vi "EZ Resistance.vi"(6 "2w/4w (F:2w)":bool, 7 "Scan List (empty)":string, 8 "error in (no error)":errorcluster, 9 "Range (7:Auto)":T2(ring)=enum."Auto", 10 "Resolution (5:Default)":T1(ring)=enum."Default", 11 "VISA Resource Name":refnum<visa-resource-name>) -> (0 "error out":errorcluster, 2 "Output Array":dbl[](array[numeric]) format="%.2f", 3 "VISA Resource Name Out":refnum<visa-resource-name>)   [LabVIEW 2017, in "Agilent 34970.lvlib"]
doc: "This VI allows you to take simple resistance measurements (either 2-wire or 4-wire)."
uses:
  <instrlib>/Agilent 34970/Agilent 34970.lvlib
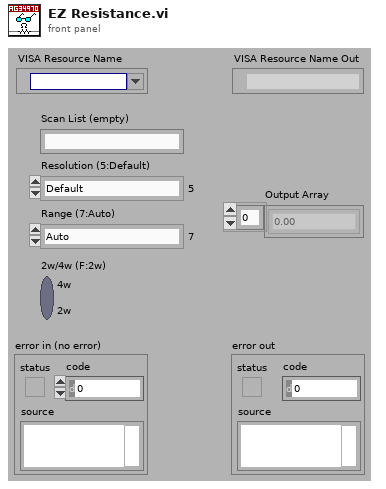
[diagram p1: front panel]
types:
  T1 = enum16{"4 1/2", "5 1/2", "6 1/2", "Least", "Highest", "Default"}
  T2 = enum16{"100 Ohm", "1 kOhm", "10 kOhm", "100 kOhm", "1 MOhm", "10 MOhm", "100 MOhm", "Auto", "Minimum", "Maximum"}
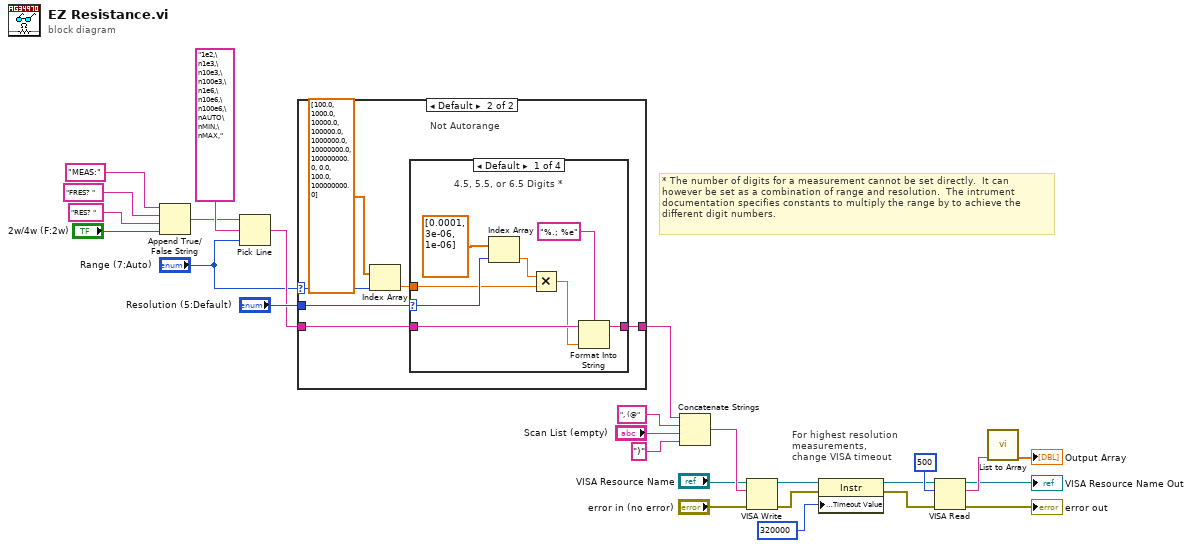
[diagram p0: block diagram]
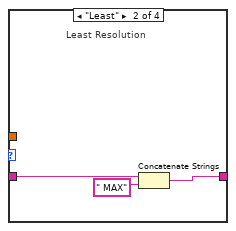
[diagram p3: hidden frame]
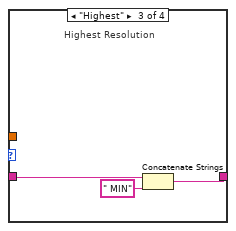
[diagram p4: hidden frame]
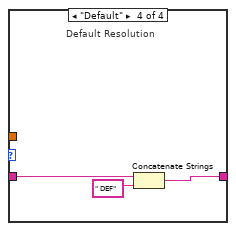
[diagram p5: hidden frame]
diagram:
  # "* The number of digits for a measurement cannot be set directly.  It can\nhowever be set as a combination of range and resolution.  The intrument\ndocumentation specifies constants to multiply the range by to achieve the\ndifferent digit numbers."
  # "For highest resolution\nmeasurements, \nchange VISA timeout"
  n1 = Append True/False String(1:"2w/4w (F:2w)", 2:"RES? ", 3:"FRES? ", 4:"MEAS:") -> (0:w14:string)
  n2 = Pick Line(string ("")=w14, multi-line string="1e2,\n1e3,\n10e3,\n100e3,\n1e6,\n10e6,\n100e6,\nAUTO\nMIN,\nMAX,", line index="Range (7:Auto)") -> (output string=w2:string)
  n3 = case shown="Default" "Range (7:Auto)" {
    selector: "Range (7:Auto)" -> [_ w33]
    tunnel: [w27 w30] -> w4
    tunnel: w2 -> [w27 w29]
    tunnel: "Resolution (5:Default)" -> [_ w31]
    frame "Auto" {
      # "Autorange"
    }
    frame Default {
      # "Not Autorange"
      n4 = Index Array(array=dbl[] [100.0, 1000.0, 10000.0, 100000.0, 1000000.0, 10000000.0, 100000000.0, 0.0, 100.0, 100000000.0], index=w33) -> (element=w28:dbl)
      n5 = case shown="Default" w31 {
        selector: w31 -> [w40 _ _ _]
        tunnel: [w34 w44 w47 w48] -> w30
        tunnel: w29 -> [w37 w43 w45 w49]
        tunnel: w28 -> [w39 _ _ _]
        frame Default {
          # "4.5, 5.5, or 6.5 Digits *"
          n6 = Index Array(array=dbl[] [0.0001, 3e-06, 1e-06], index=w40) -> (element=w38:dbl)
          n7 = Multiply(x=w38, y=w39) -> (x*y=w36:dbl)
          n8 = Format Into String(format string="%.; %e", initial string=w37, w36) -> (resulting string=w34:string)  [unwired: 1 in, 1 out]
        }
        frame "Least" {
          # "Least Resolution"
          n9 = Concatenate Strings(w43, " MAX" ("string")) -> (w44:string)
        }
        frame "Highest" {
          # "Highest Resolution"
          n10 = Concatenate Strings(w45, " MIN" ("string")) -> (w47:string)
        }
        frame "Default" {
          # "Default Resolution"
          n11 = Concatenate Strings(w49, " DEF" ("string")) -> (w48:string)
        }
      }
    }
  }
  n12 = Concatenate Strings(w4, ", (@", "Scan List (empty)", ")") -> (w10:string)
  n13 = VISA Write(VISA resource name="VISA Resource Name", write buffer=w10, error in (no error)="error in (no error)") -> (VISA resource name out=w23:refnum<visa-resource-name>, error out=w22:errorcluster)  [unwired: 1 out]
  n14 = property class="Instr"(reference=w23, error in=w22, "General Settings:Timeout Value"=u32 320000 ("Tmo Value")) -> (reference out=w20:refnum<visa-resource-name>, error out=w21:errorcluster)
  n15 = VISA Read(VISA resource name=w20, byte count=u32 500 ("byte count (0)"), error in (no error)=w21) -> (VISA resource name out=→"VISA Resource Name Out":refnum<visa-resource-name>, read buffer=w13:string, error out=→"error out":errorcluster)  [unwired: 1 out]
  n16 = call <instrlib>:"List to Array.vi"("List (empty)"=w13) -> ("Output Number Array"=→"Output Array":dbl[])  [unwired: 9 in, 1 out]
